vi "Build Description String.vi"(8 "error in (no error)":errorcluster, 11 "Visible Assertion in":refnum<class "Visible Assertion.lvclass">) -> (0 "error out":errorcluster, 2 "Description":string, 3 "Visible Assertion out":refnum<class "Visible Assertion.lvclass">)   [LabVIEW 2020, in "MacroAssert.lvlib" / "Visible Assertion.lvclass"]
doc: "Builds a string to describe what <B>Step</B> does."
uses:
  Visible Assertion.lvclass
  Visible Assertion.lvclass/Visible Assertion.ctl
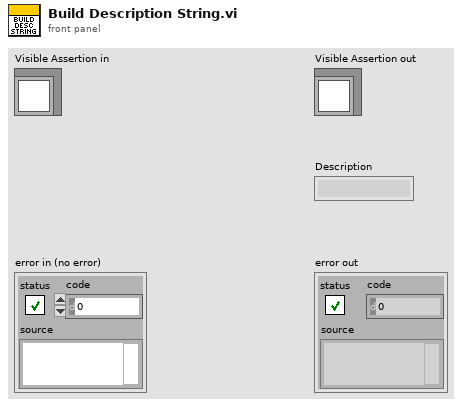
[diagram p1: front panel]
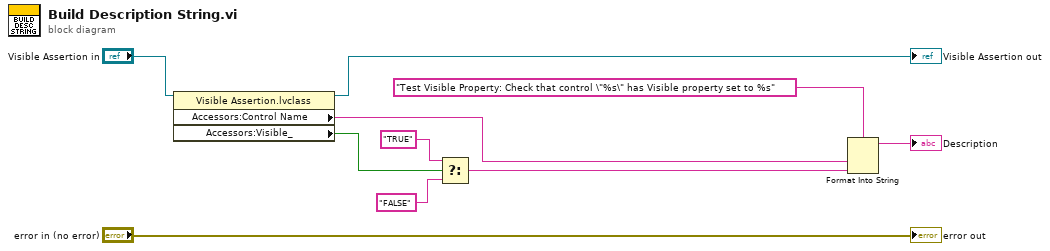
[diagram p0: block diagram]
diagram:
  n1 = property class="Visible Assertion.lvclass"(reference="Visible Assertion in") -> (reference out=→"Visible Assertion out":refnum<class "Visible Assertion.lvclass">, "Accessors:Control Name"=w2:string, "Accessors:Visible_"=w6:bool)  [unwired: 1 in, 1 out]
  n2 = Select(t="TRUE", s=w6, f="FALSE") -> (s? t:f=w3:string)
  n3 = Format Into String(format string="Test Visible Property: Check that control \"%s\" has Visible property set to %s", w2, w3) -> (resulting string=→"Description":string)  [unwired: 2 in, 1 out]
  "error out" <- "error in (no error)"
